vi "RT_readADC.vi"() -> ()   [LabVIEW 2018]
uses:
  <vilib>/Platform/TimedLoop/XDataNode/timing_clust.ctl
  <vilib>/Platform/TimedLoop/XDataNode/nitl_modes.ctl
  <vilib>/Platform/TimedLoop/XDataNode/wakeup.ctl
  <vilib>/FPGAPlugInAG/myRIO-1900/niLvFpga_Open_myRIO-1900.vi
  <vilib>/rvi/interface/common/dynamic/niFpgaDynamicAddResources.vi
  <vilib>/Utility/error.llb/Error Cluster From Error Code.vi
  <vilib>/rvi/errors/niLvFpgaAdjustHostInterfaceError.vi
  <vilib>/rvi/interface/nirviOpenFPGA/nirviOpenFPGA.xnode
  FPGA Bitfiles/ASPE2019amplifie_FPGATarget_fpgaW&RADCWritet_CjQg968FL5Q.lvbitx
  FPGA files/fpga_W&R_1ADC_W_3DAC_CLK_then_Write.vi
  <vilib>/Platform/TimedLoop/XDataNode/XDataNode.xnode
  <vilib>/rvi/interface/nirviReadWriteControl/nirviReadWriteControl.xnode
  NiFpgaLv.dll
  <vilib>/rvi/interface/Simulation/niFpgaSimulationCallBeginRW.vi
  <vilib>/Platform/TimedLoop/XDataNode/XDNodeRunTimeDep.lvlib
panel:
  out "ADC 4":dbl(graph)=-9.999542243312934
  out "ADC 3":dbl(graph)=-1.9744571768619246
  in  "CH1":bool[](array[boolean])=[FALSE, FALSE, FALSE, FALSE, FALSE, TRUE, FALSE, FALSE, FALSE, FALSE, FALSE, FALSE, FALSE, FALSE, FALSE, FALSE]
  in  "CH4":bool[](array[boolean])=[FALSE, FALSE, TRUE, TRUE, FALSE, TRUE, FALSE, FALSE, FALSE, FALSE, FALSE, FALSE, FALSE, FALSE, FALSE, FALSE]
  out "Finished Late? [i-1]":bool
  in  "us":u32=150
  out "ADC 1":dbl(graph)=-0.00701893586828814
  in  "CH3":bool[](array[boolean])=[FALSE, FALSE, FALSE, TRUE, FALSE, TRUE, FALSE, FALSE, FALSE, FALSE, FALSE, FALSE, FALSE, FALSE, FALSE, FALSE]
  in  "CH2":bool[](array[boolean])=[FALSE, FALSE, FALSE, TRUE, FALSE, TRUE, FALSE, FALSE, FALSE, FALSE, FALSE, FALSE, FALSE, FALSE, FALSE, FALSE]
  out "ADC 2":dbl(graph)=-1.9753726902360491
  in  "Stop Button":bool
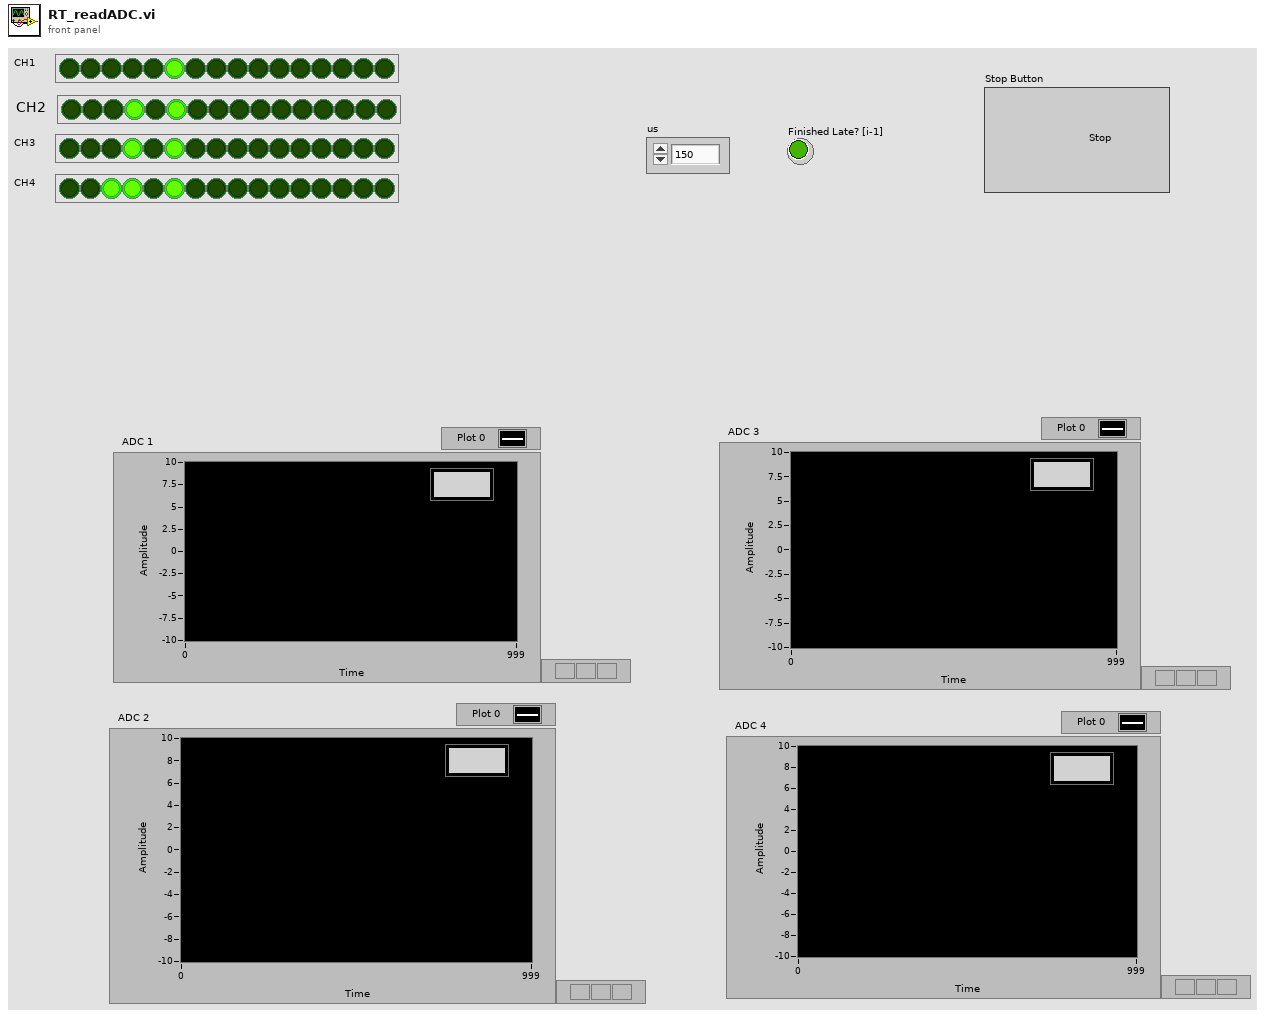
[diagram p1: front panel]
types:
  T1 = typedef "XDNodeRunTimeDep.lvlib/timing_clust.ctl" = cluster{"Expected End [f-1]":u64, "Actual End [f-1]":u64, "Finished Late? [f-1]":bool, "Expected End [i-1]":u64, "Actual End [i-1]":u64, "Finished Late? [i-1]":bool, "Expected Start [i]":u64, "Actual Start [i]":u64, "Expected Start [f]":u64, "Actual Start [f]":u64, "Source Name":string, "Structure Name":string, "Period":i64, "Deadline":i64, "Offset":i64, "Start":i64, "Priority":i32, "Timeout":i32, "Mode":T2, "Wakeup Reason":T3, "Error":errorcluster, "Source Type":string, "Secondary Source Type":string, "Global End Time":u64, "Global Start Time":u64, "Frame Duration":u64, "Iteration Duration":u64, "Assigned CPU":i32, "I/O Scan Engine Mode":u32}
  T2 = typedef "XDNodeRunTimeDep.lvlib/nitl_modes.ctl" = enum32{"No Change", "Process missed periods, maintain original phase", "Discard missed periods, maintain original phase", "Process missed periods, ignore original phase", "Discard missed periods, ignore original phase"}
  T3 = typedef "XDNodeRunTimeDep.lvlib/wakeup.ctl" = enum32{"Normal", "Aborted", "Asynchronous wakeup", "Timing source error", "Timed loop error", "Timeout"}
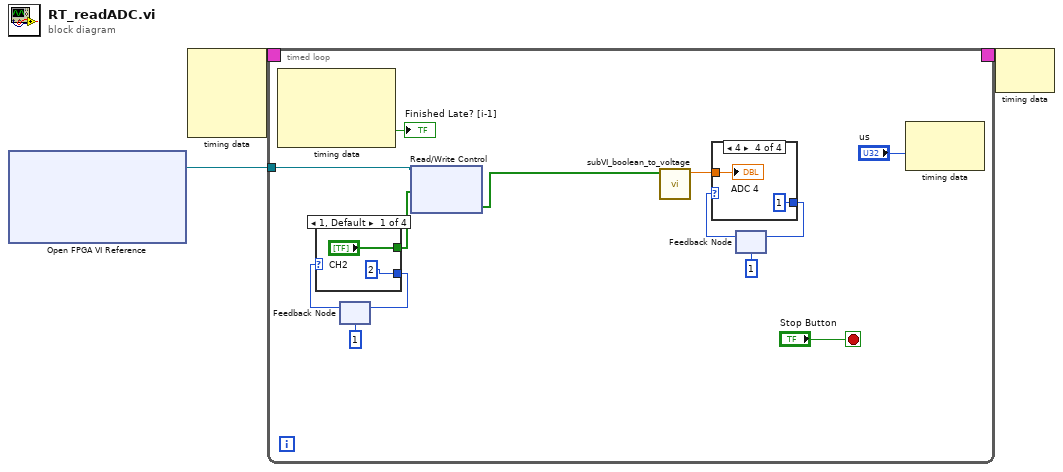
[diagram p0: block diagram]
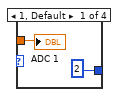
[diagram p2: hidden frame]
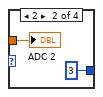
[diagram p3: hidden frame]
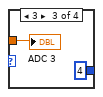
[diagram p4: hidden frame]
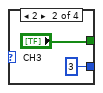
[diagram p5: hidden frame]
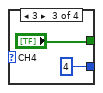
[diagram p6: hidden frame]
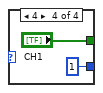
[diagram p7: hidden frame]
diagram:
  n1 = xnode "Open FPGA VI Reference"() -> ("FPGA VI Reference Out"=w3:refnum<k20>)  [unwired: 2 in, 1 out]
  n2 = node-c288() -> (w2:T1)  [unwired: 4 in]
  n3 = timed-loop {
    tunnel: w3 -> [w16]
    timing: w2 -> [_]
    timing-out: [_] -> w1
    stop <- "Stop Button" stop-if-true
    n4 = node-c288() -> (→"Finished Late? [i-1]":bool)  [unwired: 1 in, 3 out]
    n5 = feedback #1(1) -> (w14:i32)
    n6 = case shown="1, Default" w14 {
      tunnel: ["CH2" "CH3" "CH4" "CH1"] -> w11
      tunnel: [2 3 4 1] -> w12
      frame 1, Default {
      }
      frame 2 {
      }
      frame 3 {
      }
      frame 4 {
      }
    }
    n7 = feedback-in #1(w12) -> ()
    n8 = xnode "Read/Write Control"("FPGA VI Reference In"=w16, "ADC write"=w11) -> ("ADC read"=w4:bool[])  [unwired: 1 in, 2 out]
    n9 = call "subVI_boolean_to_voltage.vi"("ADC read"=w4) -> ("V"=w7:dbl)  [unwired: 10 in]
    n10 = feedback #2(1) -> (w10:i32)
    n11 = case shown="4" w10 {
      tunnel: [2 3 4 1] -> w8
      tunnel: w7 -> [w22 w24 w26 w28]
      frame 1, Default {
        "ADC 1" <- w22
      }
      frame 2 {
        "ADC 2" <- w24
      }
      frame 3 {
        "ADC 3" <- w26
      }
      frame 4 {
        "ADC 4" <- w28
      }
    }
    n12 = feedback-in #2(w8) -> ()
    n13 = node-c288("us") -> ()  [unwired: 1 in, 1 out]
  }
  n14 = node-c288(w1) -> ()  [unwired: 1 out]
